vi "Login.vi"(6 "error in (no error)":errorcluster caption="에러 입력(에러 없음)") -> (0 "error out":errorcluster caption="에러 출력", 2 "State":T2)   [LabVIEW 2019]
uses:
  controller/idForm.ctl
  controller/passwordForm.ctl
  controller/signInBtn.ctl
  03_Home/controller/pannelState.ctl
  03_Home/controller/exitBtn.ctl
  <vilib>/Utility/miscctls.llb/LVPointTypeDef.ctl
  globalValue.vi
panel:
  in  "Exit Button":T1
  in  "signUp":bool
  in  "findPw":bool
  in  "findId":bool
  in  "loginBtn":T3
  in  "password":T4
  in  "id":T5
  # "|"
  # "계정이 없으신가요?"
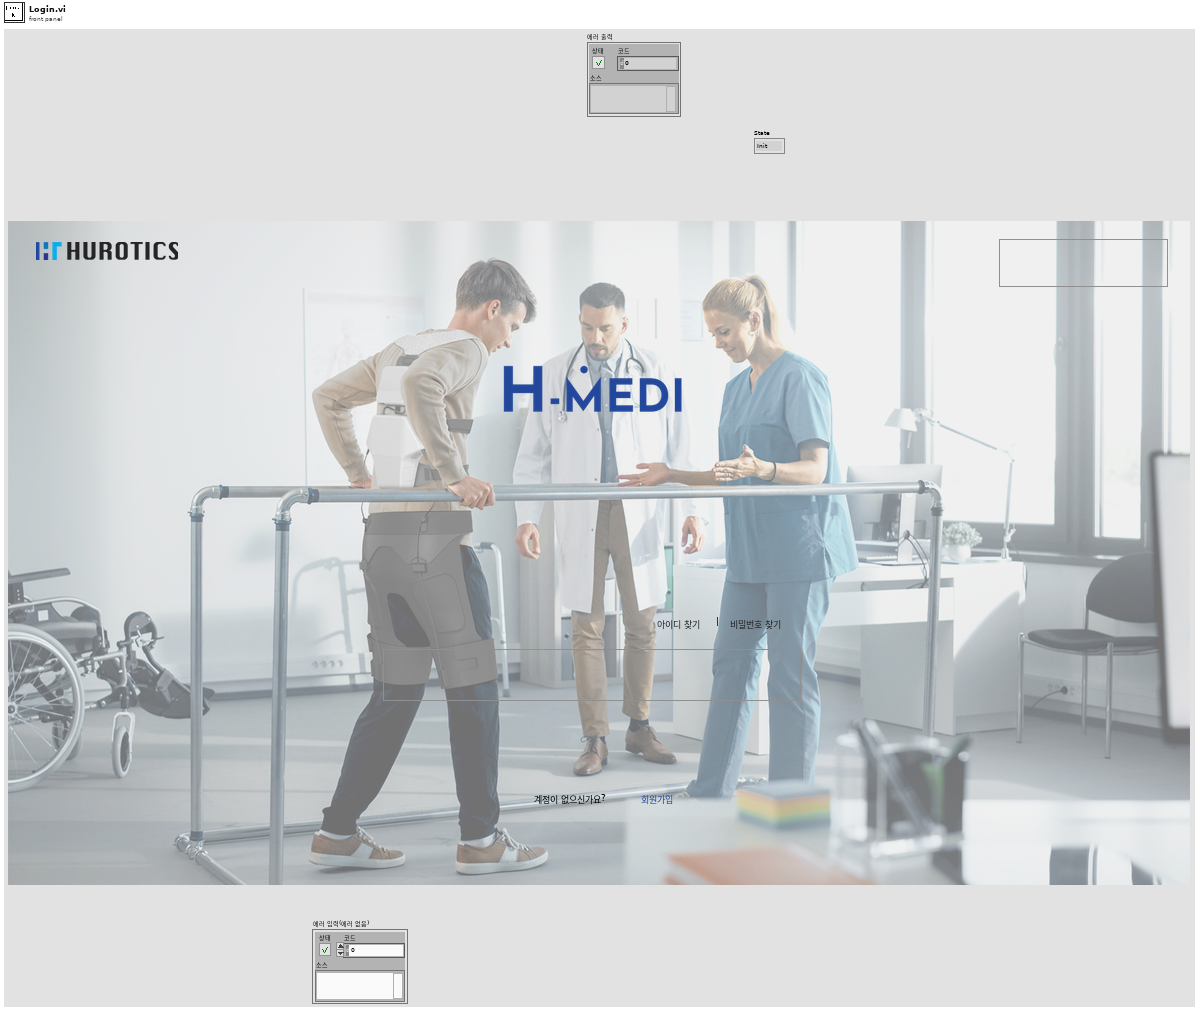
[diagram p1: front panel]
types:
  T1 = typedef "exitBtn.ctl" = bool
  T2 = typedef "pannelState.ctl" = enum16{"Init", "LogIn", "SignUpView", "Home", "Management_patientList", "Management_patientTrashtList", "Management_patientCreate", "Management_patientUpdate", "Management_patientTraining", "Management_patientTrainingDetail", "H-MEDI PatientList", "H-MEDI HardwareCtl", "Adjust", "FineTuning", "UserList", "UserDetail", "Exit"}
  T3 = typedef "signInBtn.ctl" = bool
  T4 = typedef "passwordForm.ctl" = string
  T5 = typedef "idForm.ctl" = string
  T6 = typedef "LVPointTypeDef.ctl" = cluster{"Horizontal":i16, "Vertical":i16}
  T7 = enum16{"connection", "create", "read", "update", "delete", "close"}
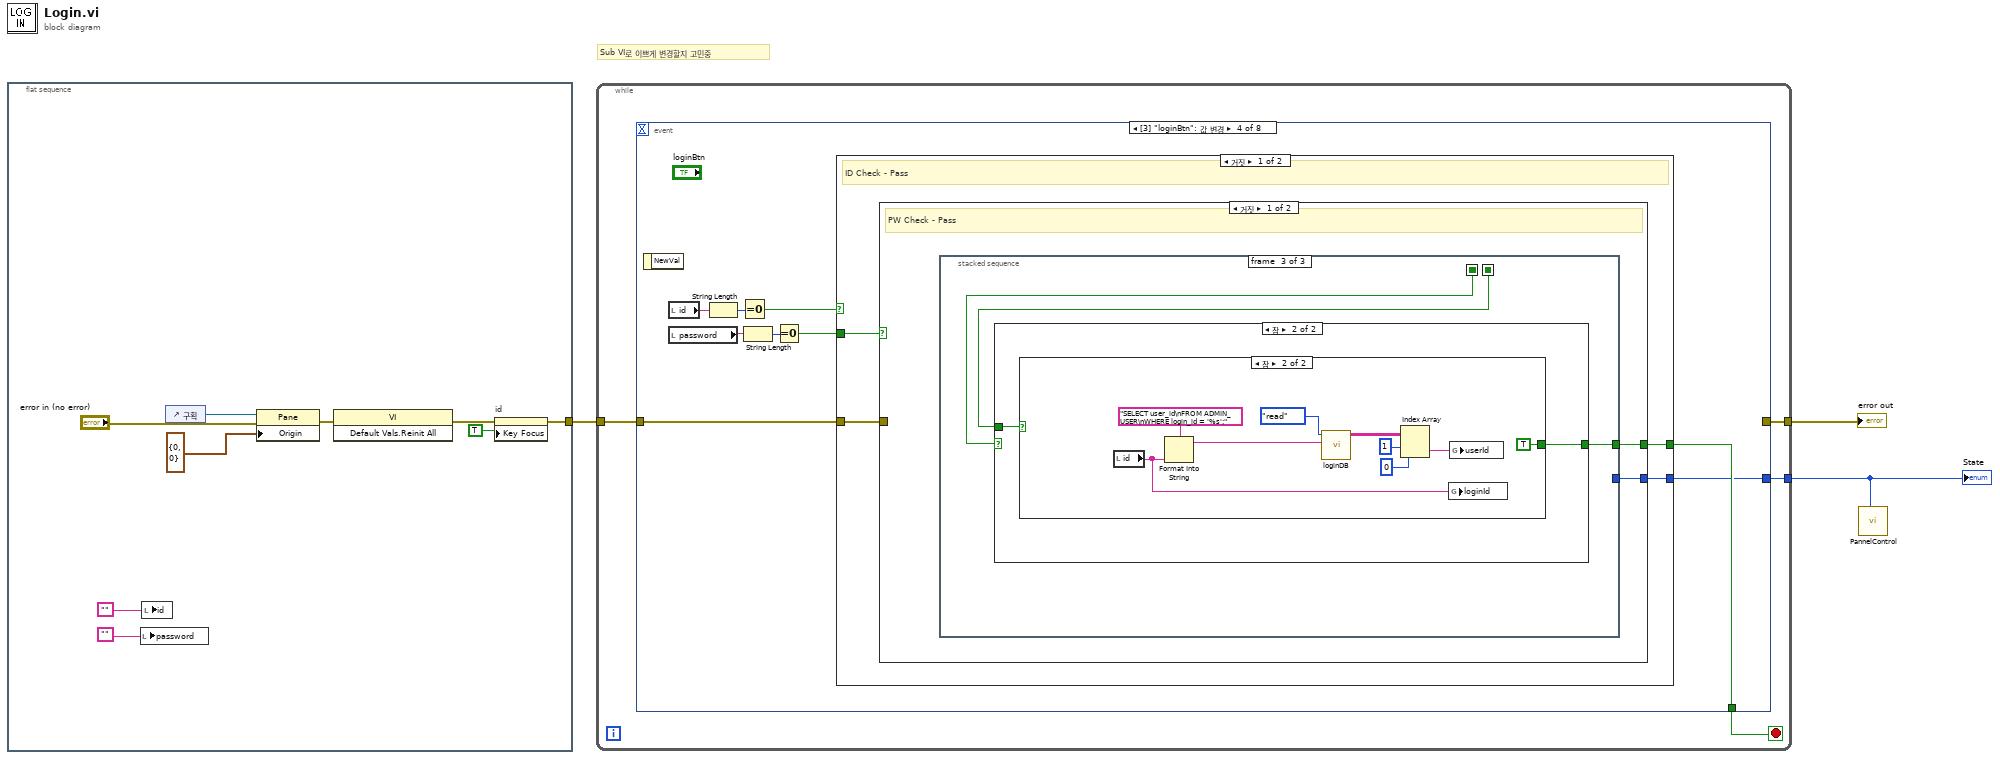
[diagram p0: block diagram]
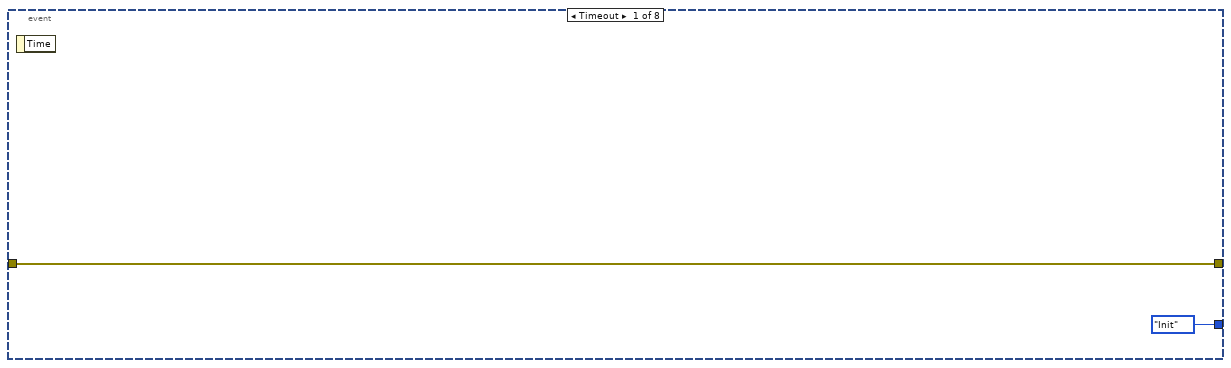
[diagram p2: hidden frame]
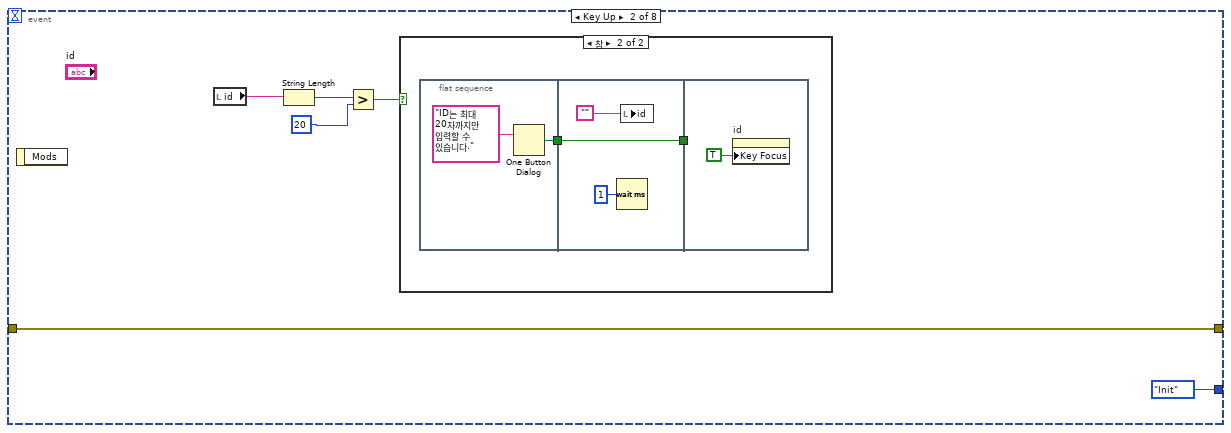
[diagram p3: hidden frame]
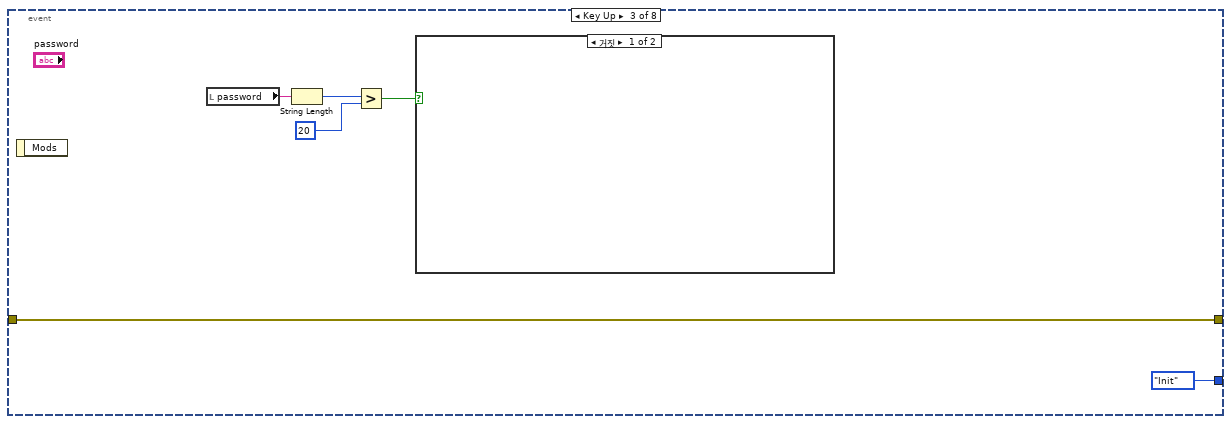
[diagram p5: hidden frame]
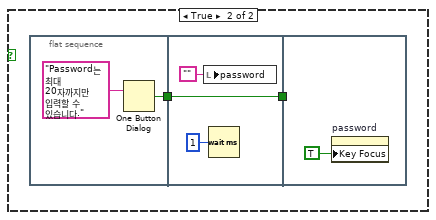
[diagram p6: hidden frame]
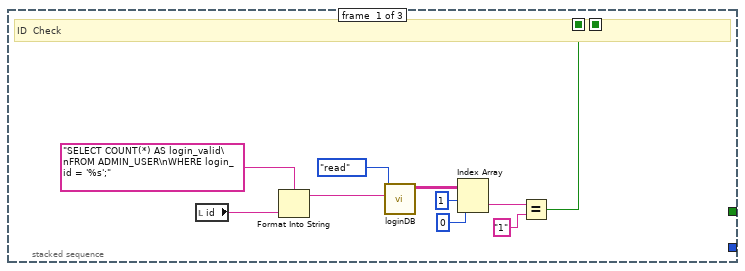
[diagram p7: hidden frame]
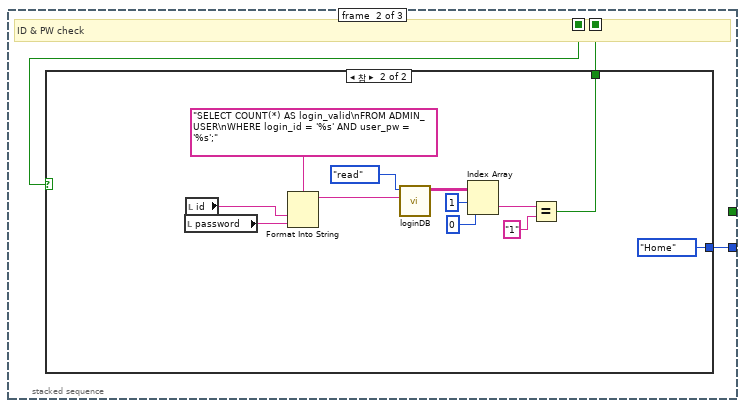
[diagram p8: hidden frame]
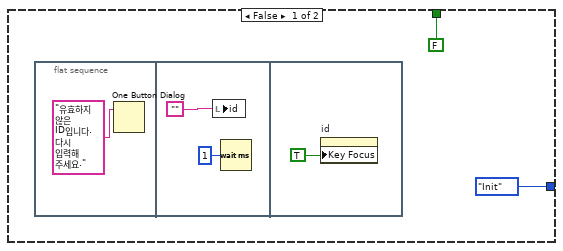
[diagram p9: hidden frame]
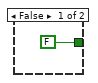
[diagram p10: hidden frame]
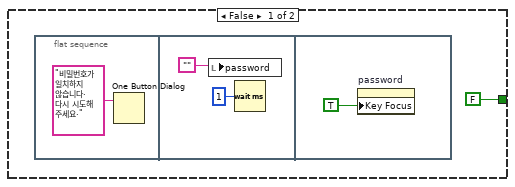
[diagram p11: hidden frame]
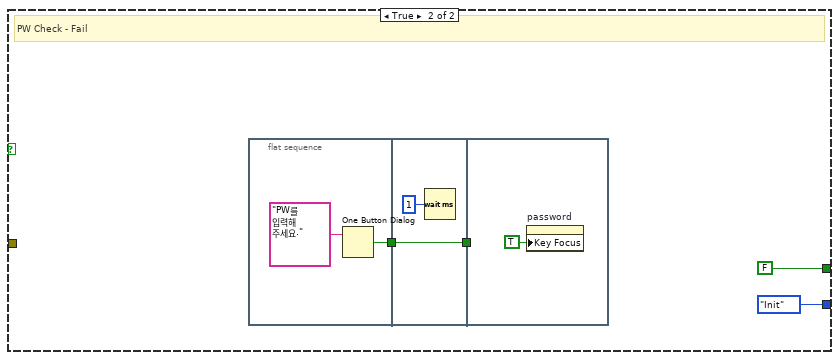
[diagram p12: hidden frame]
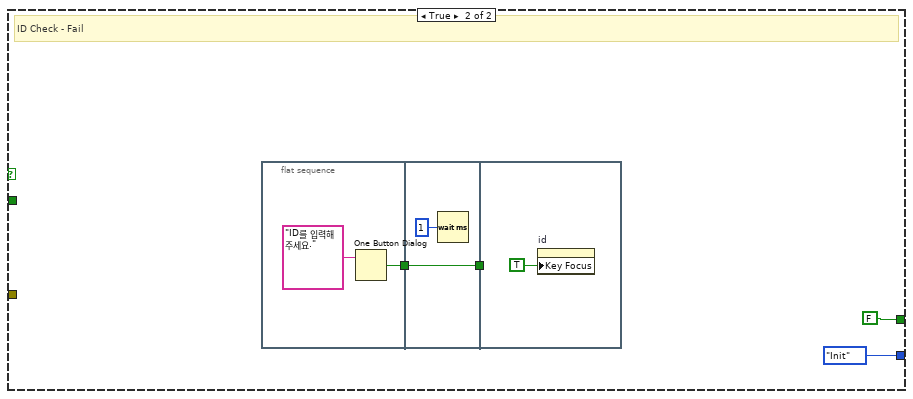
[diagram p13: hidden frame]
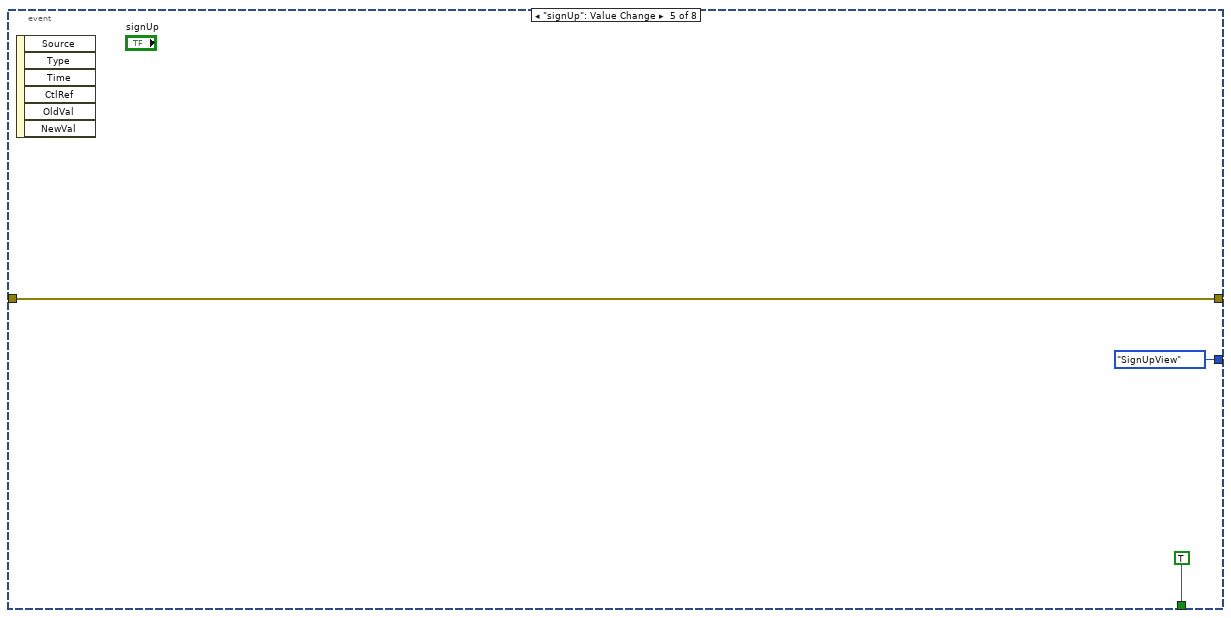
[diagram p14: hidden frame]
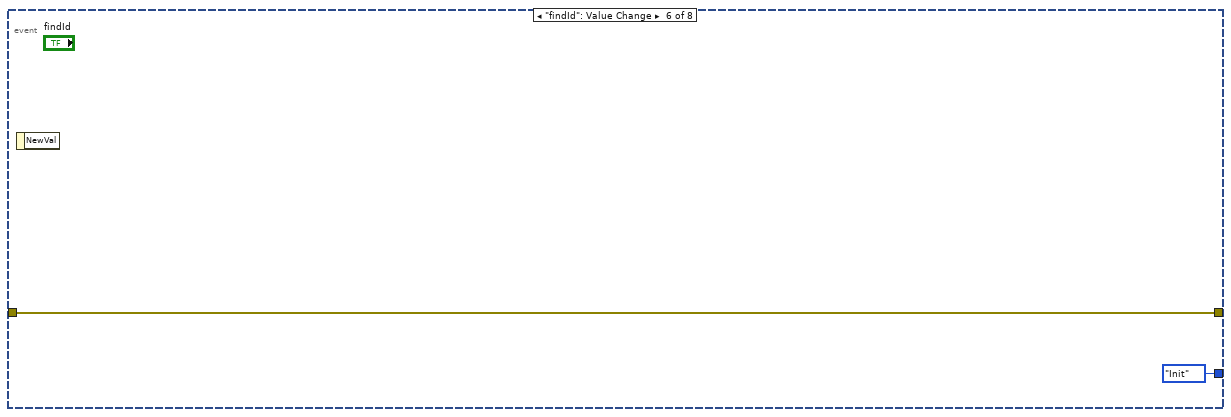
[diagram p15: hidden frame]
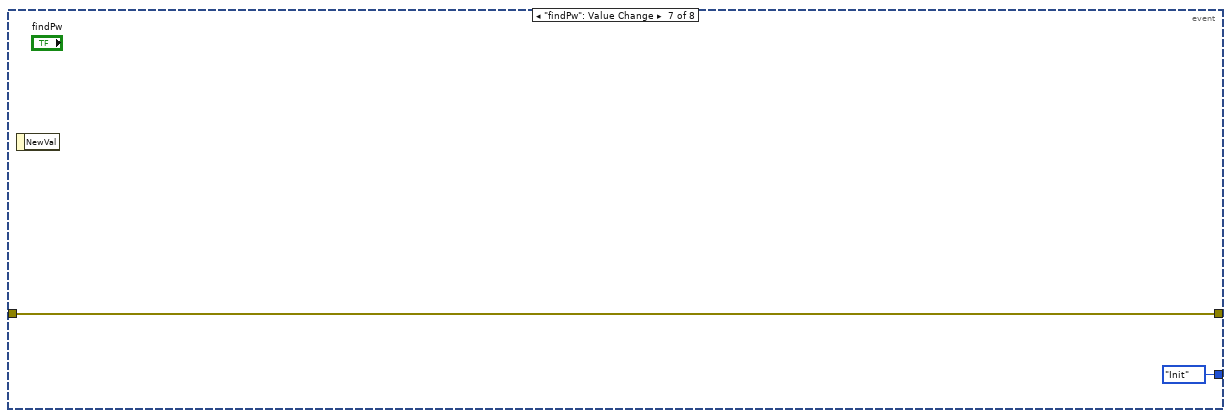
[diagram p16: hidden frame]
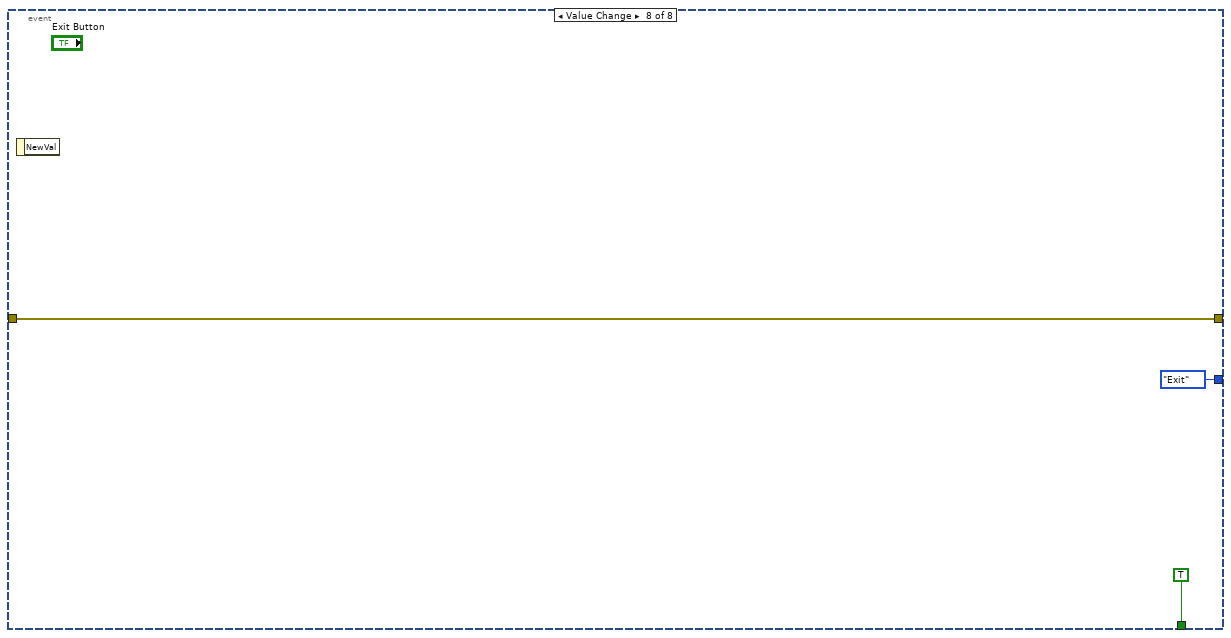
[diagram p17: hidden frame]
diagram:
  # "Sub VI로 이쁘게 변경할지 고민중"
  n1 = flat-sequence {
    tunnel: [w4] -> w2
    frame #0 {
      n2 = local write "password"("") -> ()
      n3 = local write "id"("") -> ()
      n4 = control-ref of="구획"() -> (w11:refnum<vi>)
      n5 = property class="Pane"(reference=w11, error in="error in (no error)", "Origin"=T6 {"Horizontal"=0, "Vertical"=0} ("원점")) -> (error out=w10:errorcluster)  [unwired: 1 out]
      n6 = invoke class="VI" method="Default Vals.Reinit All"(error in=w10) -> (error out=w6:errorcluster)  [unwired: 2 in, 2 out]
      n7 = property on="id" class="Str (엄격한)"(error in=w6, "Key Focus"=TRUE ("키 포커스")) -> (error out=w4:errorcluster)  [unwired: 1 in, 1 out]
    }
  }
  n8 = while {
    tunnel: w2 -> [w15]
    tunnel: [w14] -> w3
    tunnel: [w13] -> w1
    stop <- w16 stop-if-true
    n9 = event shown="[3] \"loginBtn\": 값 변경" {
      selector: _ -> [_ _ _ _ _ _ _ _]
      dyn-events: _ -> [_ _ _ _ _ _ _ _]
      timeout: _ -> [_ _ _ _ _ _ _ _]
      tunnel: [_ _ _ w51 TRUE _ _ TRUE] -> w16
      tunnel: w15 -> [w17 w19 w33 w52 w131 w134 w136 w138]
      tunnel: [pannelState."Init" ("State") pannelState."Init" ("State") pannelState."Init" ("State") w50 pannelState."SignUpView" ("State") pannelState."Init" ("State") pannelState."Init" ("State") pannelState."Exit" ("State")] -> w14
      tunnel: [w17 w19 w33 _ w131 w134 w136 w138] -> w13
      event Timeout {
        n10 = event-data() -> ()  [unwired: 1 in, 1 out]
      }
      event Key Up {
        n11 = event-data() -> ()  [unwired: 1 in, 1 out]
        n12 = local read "id"() -> (w22:T5)
        n13 = String Length(string=w22) -> (length=w24:i32)
        n14 = Greater?(x=w24, y=20) -> (0:w23:bool)
        n15 = case shown="참" w23 {
          frame False {
          }
          frame True {
            n16 = flat-sequence {
              tunnel: [w27] -> w26
              tunnel: w26 -> [w31]
              tunnel: [w31] -> w25
              tunnel: w25 -> [_]
              frame #0 {
                n17 = One Button Dialog(message="ID는 최대 20자까지만 입력할 수 있습니다." ("메시지")) -> (true=w27:bool)  [unwired: 1 in]
              }
              frame #1 {
                n18 = Wait (ms)(milliseconds to wait=u32 1 ("대기 시간 (ms)")) -> ()  [unwired: 1 out]
                n19 = local write "id"("") -> ()
              }
              frame #2 {
                n20 = property on="id" class="Str (엄격한)"("Key Focus"=TRUE ("키 포커스")) -> ()  [unwired: 2 in, 2 out]
              }
            }
          }
        }
      }
      event Key Up {
        n21 = event-data() -> ()  [unwired: 1 in, 1 out]
        n22 = local read "password"() -> (w35:T4)
        n23 = String Length(string=w35) -> (length=w38:i32)
        n24 = Greater?(x=w38, y=20) -> (0:w36:bool)
        n25 = case shown="거짓" w36 {
          frame False {
          }
          frame True {
            n26 = flat-sequence {
              tunnel: [w41] -> w40
              tunnel: w40 -> [w45]
              tunnel: [w45] -> w39
              tunnel: w39 -> [_]
              frame #0 {
                n27 = One Button Dialog(message="Password는 최대 20자까지만 입력할 수 있습니다." ("메시지")) -> (true=w41:bool)  [unwired: 1 in]
              }
              frame #1 {
                n28 = local write "password"("") -> ()
                n29 = Wait (ms)(milliseconds to wait=u32 1 ("대기 시간 (ms)")) -> ()  [unwired: 1 out]
              }
              frame #2 {
                n30 = property on="password" class="Str (엄격한)"("Key Focus"=TRUE ("키 포커스")) -> ()  [unwired: 2 in, 2 out]
              }
            }
          }
        }
      }
      event Value Change {
        n31 = event-data() -> ()  [unwired: 1 in, 1 out]
        n32 = local read "id"() -> (w55:T5)
        n33 = local read "password"() -> (w48:T4)
        n34 = String Length(string=w55) -> (length=w54:i32)
        n35 = Equal To 0?(x=w54) -> (x = 0?=w53:bool)
        n36 = String Length(string=w48) -> (length=w49:i32)
        n37 = Equal To 0?(x=w49) -> (x = 0?=w47:bool)
        n38 = case shown="거짓" w53 {
          tunnel: w52 -> [w59 _]
          tunnel: [w57 FALSE] -> w51
          tunnel: [w58 pannelState."Init" ("State")] -> w50
          tunnel: w47 -> [w56 _]
          frame False {
            # "ID Check - Pass"
            n39 = case shown="거짓" w56 {
              tunnel: w59 -> [_ _]
              tunnel: [w61 pannelState."Init" ("State")] -> w58
              tunnel: [w60 FALSE] -> w57
              frame False {
                # "PW Check - Pass"
                n40 = stacked-sequence {
                  seq-local: [w62 _ _] -> [_ w74 w95]
                  seq-local: [_ w73 _] -> [_ _ w94]
                  tunnel: [_ w72 _] -> w61
                  tunnel: [_ _ w93] -> w60
                  frame #0 {
                    # "ID  Check"
                    n41 = local read "id"() -> (w63:T5)
                    n42 = Format Into String(format string="SELECT COUNT(*) AS login_valid\nFROM ADMIN_USER\nWHERE login_id = '%s';", w63) -> (resulting string=w69:string)  [unwired: 2 in, 1 out]
                    n43 = call "loginDB.vi"("Query"=w69, "State"=T7."read") -> ("Result Set"=w70:string[][])  [unwired: 7 in, 1 out]
                    n44 = Index Array(array=w70, index (row)=1 ("인덱스 (행)"), index (col)=0 ("비활성화된 인덱스 (열)")) -> (element=w67:string)
                    n45 = Equal?(x=w67, y="1") -> (x = y?=w62:bool)
                  }
                  frame #1 {
                    # "ID & PW check"
                    n46 = case shown="참" w74 {
                      tunnel: [pannelState."Init" ("State") pannelState."Home" ("State")] -> w72
                      tunnel: [FALSE w81] -> w73
                      frame False {
                        n47 = flat-sequence {
                          frame #0 {
                            n48 = One Button Dialog(message="유효하지 않은 ID입니다. 다시 입력해 주세요." ("메시지")) -> ()  [unwired: 1 in, 1 out]
                          }
                          frame #1 {
                            n49 = local write "id"("") -> ()
                            n50 = Wait (ms)(milliseconds to wait=u32 1 ("대기 시간 (ms)")) -> ()  [unwired: 1 out]
                          }
                          frame #2 {
                            n51 = property on="id" class="Str (엄격한)"("Key Focus"=TRUE ("키 포커스")) -> ()  [unwired: 2 in, 2 out]
                          }
                        }
                      }
                      frame True {
                        n52 = local read "password"() -> (w87:T4)
                        n53 = local read "id"() -> (w82:T5)
                        n54 = Format Into String(format string="SELECT COUNT(*) AS login_valid\nFROM ADMIN_USER\nWHERE login_id = '%s' AND user_pw = '%s';", w82, w87) -> (resulting string=w85:string)  [unwired: 2 in, 1 out]
                        n55 = call "loginDB.vi"("Query"=w85, "State"=T7."read") -> ("Result Set"=w84:string[][])  [unwired: 7 in, 1 out]
                        n56 = Index Array(array=w84, index (row)=1 ("인덱스 (행)"), index (col)=0 ("비활성화된 인덱스 (열)")) -> (element=w91:string)
                        n57 = Equal?(x=w91, y="1") -> (x = y?=w81:bool)
                      }
                    }
                  }
                  frame #2 {
                    n58 = case shown="참" w95 {
                      tunnel: w94 -> [_ w98]
                      tunnel: [FALSE w97] -> w93
                      frame False {
                      }
                      frame True {
                        n59 = case shown="참" w98 {
                          tunnel: [FALSE TRUE] -> w97
                          frame False {
                            n60 = flat-sequence {
                              frame #0 {
                                n61 = One Button Dialog(message="비밀번호가 일치하지 않습니다. 다시 시도해 주세요." ("메시지")) -> ()  [unwired: 1 in, 1 out]
                              }
                              frame #1 {
                                n62 = local write "password"("") -> ()
                                n63 = Wait (ms)(milliseconds to wait=u32 1 ("대기 시간 (ms)")) -> ()  [unwired: 1 out]
                              }
                              frame #2 {
                                n64 = property on="password" class="Str (엄격한)"("Key Focus"=TRUE ("키 포커스")) -> ()  [unwired: 2 in, 2 out]
                              }
                            }
                          }
                          frame True {
                            n65 = local read "id"() -> (w105:T5)
                            n66 = Format Into String(format string="SELECT user_id\nFROM ADMIN_USER\nWHERE login_id = '%s';", w105) -> (resulting string=w106:string)  [unwired: 2 in, 1 out]
                            n67 = call "loginDB.vi"("Query"=w106, "State"=T7."read") -> ("Result Set"=w109:string[][])  [unwired: 7 in, 1 out]
                            n68 = Index Array(array=w109, index (row)=1 ("인덱스 (행)"), index (col)=0 ("비활성화된 인덱스 (열)")) -> (element=w108:string)
                            n69 = global write "globalValue.vi" "loginId"(w105) -> ()
                            n70 = global write "globalValue.vi" "userId"(w108) -> ()
                          }
                        }
                      }
                    }
                  }
                }
              }
              frame True {
                # "PW Check - Fail"
                n71 = flat-sequence {
                  tunnel: [w117] -> w114
                  tunnel: w114 -> [w120]
                  tunnel: [w120] -> w113
                  tunnel: w113 -> [_]
                  frame #0 {
                    n72 = One Button Dialog(message="PW를 입력해 주세요.") -> (true=w117:bool)  [unwired: 1 in]
                  }
                  frame #1 {
                    n73 = Wait (ms)(milliseconds to wait=u32 1 ("대기 시간 (ms)")) -> ()  [unwired: 1 out]
                  }
                  frame #2 {
                    n74 = property on="password" class="Str (엄격한)"("Key Focus"=TRUE ("키 포커스")) -> ()  [unwired: 2 in, 2 out]
                  }
                }
              }
            }
          }
          frame True {
            # "ID Check - Fail"
            n75 = flat-sequence {
              tunnel: [w126] -> w125
              tunnel: w125 -> [w129]
              tunnel: [w129] -> w124
              tunnel: w124 -> [_]
              frame #0 {
                n76 = One Button Dialog(message="ID를 입력해 주세요.") -> (true=w126:bool)  [unwired: 1 in]
              }
              frame #1 {
                n77 = Wait (ms)(milliseconds to wait=u32 1 ("대기 시간 (ms)")) -> ()  [unwired: 1 out]
              }
              frame #2 {
                n78 = property on="id" class="Str (엄격한)"("Key Focus"=TRUE ("키 포커스")) -> ()  [unwired: 2 in, 2 out]
              }
            }
          }
        }
      }
      event "signUp": Value Change {
        n79 = event-data() -> ()  [unwired: 1 in, 6 out]
      }
      event "findId": Value Change {
        n80 = event-data() -> ()  [unwired: 1 in, 1 out]
      }
      event "findPw": Value Change {
        n81 = event-data() -> ()  [unwired: 1 in, 1 out]
      }
      event Value Change {
        n82 = event-data() -> ()  [unwired: 1 in, 1 out]
      }
    }
  }
  "error out" <- w1
  "State" <- w3
  n83 = call "PannelControl.vi"("State"=w3) -> ()  [unwired: 10 in, 1 out]
